vi "Write Roles.vi"(8 "error in (no error)":errorcluster, 10 "Roles":T1, 11 "PreparePenaltyAllyPlayVSS in":refnum<class "PreparePenaltyAllyPlayVSS.lvclass">) -> (0 "error out":errorcluster, 3 "PreparePenaltyAllyPlayVSS out":refnum<class "PreparePenaltyAllyPlayVSS.lvclass">)   [LabVIEW 2023, in "PreparePenaltyAllyPlayVSS.lvclass"]
uses:
  PreparePenaltyAllyPlayVSS.lvclass
  HaltRole_class/HaltRole.lvclass
  AttackerAimGoalRoleVSS_class/AttackerAimGoalRoleVSS.lvclass
  PreparePenaltyAllyPlayVSS.lvclass/PreparePenaltyAllyPlayVSS.ctl
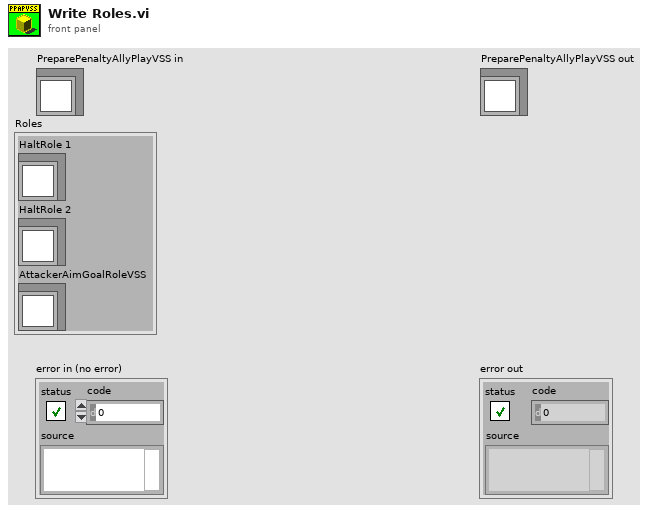
[diagram p1: front panel]
types:
  T1 = cluster{"HaltRole 1":refnum<class "HaltRole.lvclass">, "HaltRole 2":refnum<class "HaltRole.lvclass">, "AttackerAimGoalRoleVSS":refnum<class "AttackerAimGoalRoleVSS.lvclass">}
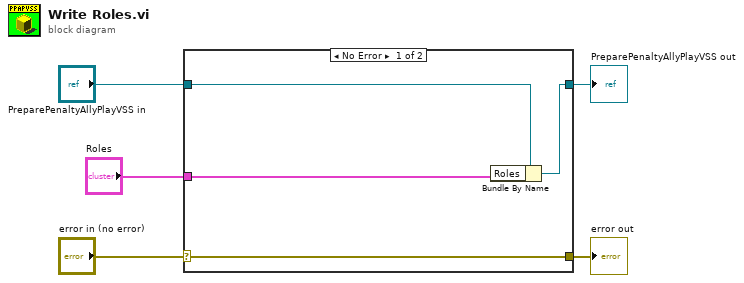
[diagram p0: block diagram]
diagram:
  n1 = case shown="No Error" "error in (no error)" {
    selector: "error in (no error)" -> [w9 w10]
    tunnel: [w9 w10] -> w4
    tunnel: [w7 w11] -> w2
    tunnel: "PreparePenaltyAllyPlayVSS in" -> [w8 w11]
    tunnel: "Roles" -> [w6 _]
    frame No Error {
      n2 = Bundle By Name(cluster=w8, "Roles"=w6) -> (w7:refnum<class "PreparePenaltyAllyPlayVSS.lvclass">)
    }
    frame Error {
    }
  }
  "error out" <- w4
  "PreparePenaltyAllyPlayVSS out" <- w2
